vi "needTochangeToStaging.vi"(11 "output cluster":T1={"Main interlock"=TRUE, "Flow Switch 1"=TRUE, "Flow Switch 2"=TRUE, "Power Supply ok"=FALSE, "on"=TRUE, "staging"=TRUE, "undulator"=FALSE, "VOLTAGE"=0.0, "CURRENT"=0.0, "curent set"=0}) -> (2 "change to staging":bool, 3 "output cluster 2":T1={"Main interlock"=TRUE, "Flow Switch 1"=TRUE, "Flow Switch 2"=TRUE, "Power Supply ok"=FALSE, "on"=TRUE, "staging"=TRUE, "undulator"=FALSE, "VOLTAGE"=0.0, "CURRENT"=0.0, "curent set"=0})   [LabVIEW 2013]
uses:
  MagnetCluster.ctl
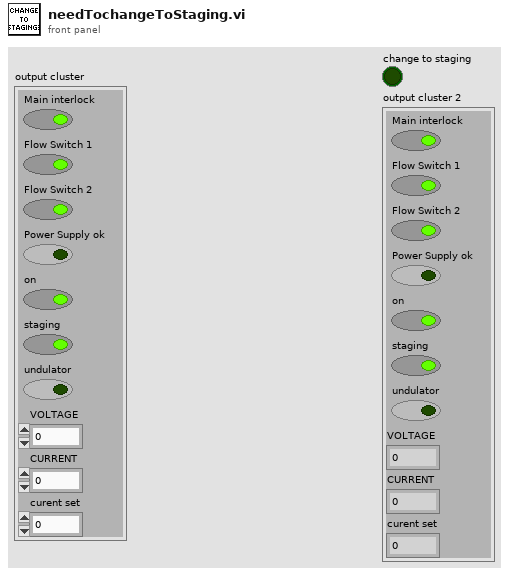
[diagram p1: front panel]
types:
  T1 = typedef "MagnetCluster.ctl" = cluster{"Main interlock":bool, "Flow Switch 1":bool, "Flow Switch 2":bool, "Power Supply ok":bool, "on":bool, "staging":bool, "undulator":bool, "VOLTAGE":dbl, "CURRENT":dbl, "curent set":u16}
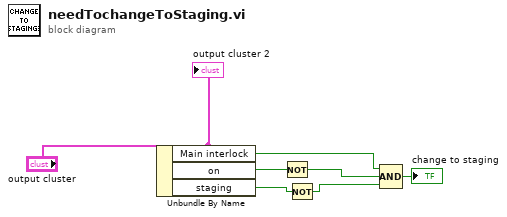
[diagram p0: block diagram]
diagram:
  n1 = Unbundle By Name("output cluster") -> ("Main interlock"=w5:bool, "on"=w6:bool, "staging"=w2:bool)
  n2 = Not(x=w6) -> (.not. x?=w4:bool)
  n3 = Not(x=w2) -> (.not. x?=w1:bool)
  n4 = Compound Arithmetic op=AND(w5, w4, w1) -> (→"change to staging":bool)
  "output cluster 2" <- "output cluster"
